vi "PQprepare.vi"(4 "paramTypes":u64[](array[numeric]), 6 "nParams":u64, 8 "error in (no error)":errorcluster, 9 "query":string, 10 "stmtName":string, 11 "conn":u64) -> (0 "error out":errorcluster, 2 "res":u64, 3 "conn_out":u64)   [LabVIEW 2019, in "libpqlv64.lvlib"]
doc: "Submits a request to create a prepared statement with the given parameters, and waits for completion.\n\nhttp://www.postgresql.org/docs/8.1/interactive/libpq-exec.html"
uses:
  libpqlv64.lvlib
  libpq.dll
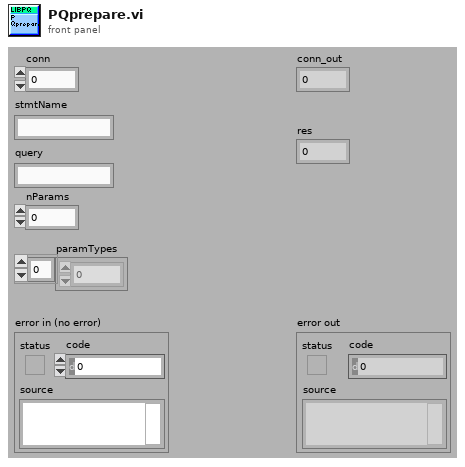
[diagram p1: front panel]
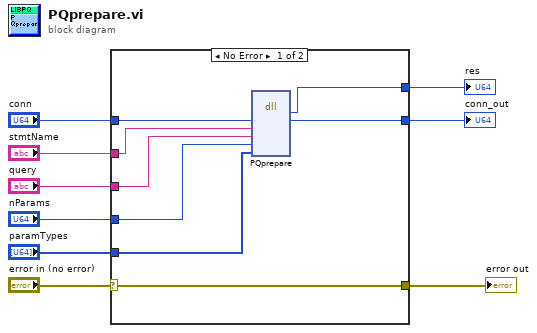
[diagram p0: block diagram]
diagram:
  n1 = case shown="No Error" "error in (no error)" {
    selector: "error in (no error)" -> [w17 w19]
    tunnel: [w17 w19] -> w8
    tunnel: [w16 _] -> w7
    tunnel: "stmtName" -> [w15 _]
    tunnel: "query" -> [w14 _]
    tunnel: "nParams" -> [w13 _]
    tunnel: "paramTypes" -> [w12 _]
    tunnel: "conn" -> [w11 w18]
    tunnel: [w10 w18] -> w1
    frame No Error {
      n2 = dll-call lib="libpq.*" fn="PQprepare"("conn"=w11, "stmtName"=w15, "query"=w14, "nParams"=w13, "paramTypes"=w12) -> ("res"=w16:u64, "conn"=w10:u64)  [unwired: 7 in, 2 out]
    }
    frame Error {
    }
  }
  "res" <- w7
  "error out" <- w8
  "conn_out" <- w1
